vi "AMZ_S3_APIHLP_Parse NotificationConfiguration.vi"(8 "error in (no error)":errorcluster, 10 "Response body":string) -> (0 "error out":errorcluster, 3 "NotificationConfiguration":T1)   [LabVIEW 2015, in "LV Interface for Amazon S3.lvlib"]
uses:
  LV Interface for Amazon S3.lvlib
  Typedefs/AMZ_S3_NotificationConfiguration.ctl
  Typedefs/AMZ_S3_CompleteTopicConfiguration.ctl
  Typedefs/AMZ_S3_Event.ctl
  Typedefs/AMZ_S3_FilterRule.ctl
  Typedefs/AMZ_S3_CloudFunctionConfiguration.ctl
  Typedefs/AMZ_S3_QueueConfiguration.ctl
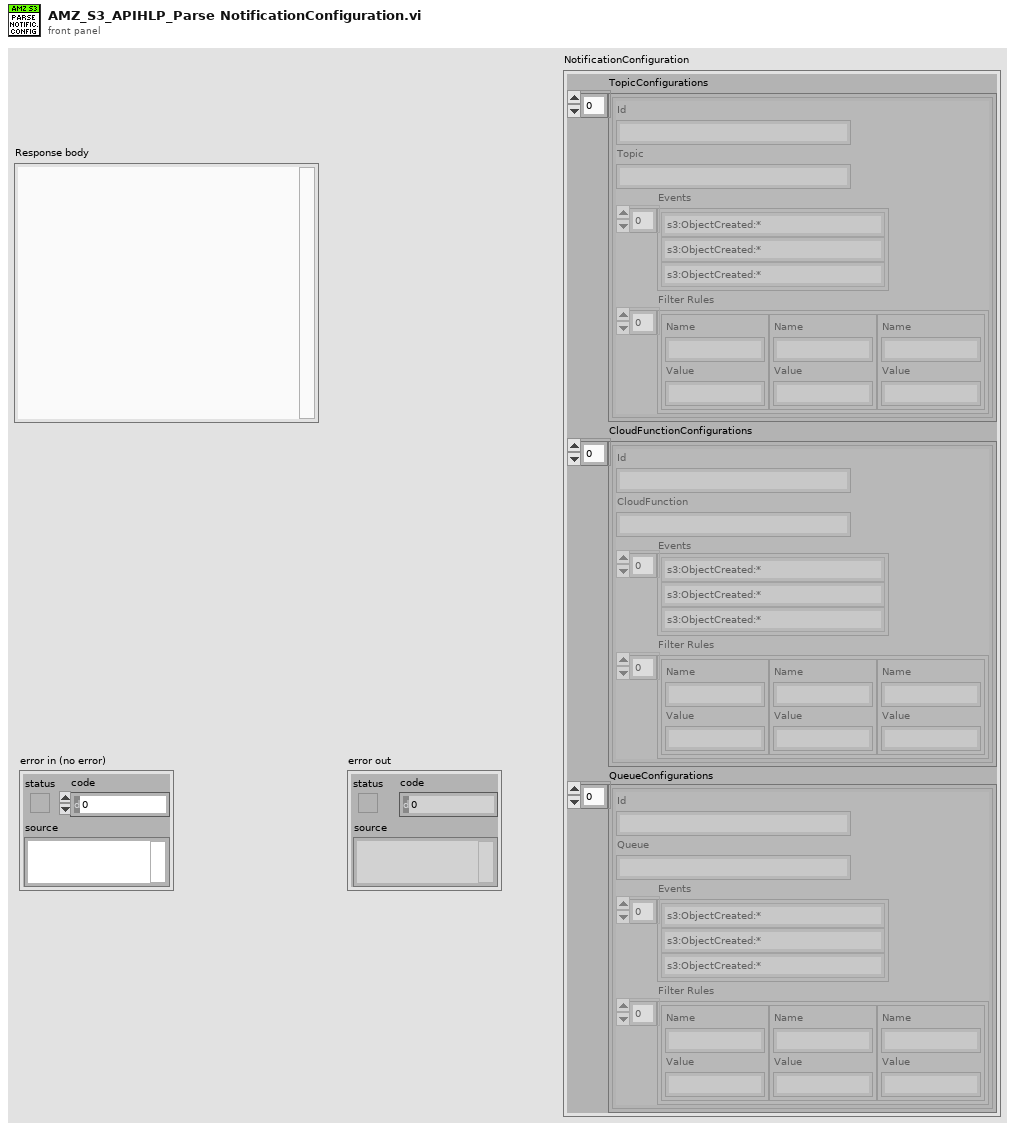
[diagram p1: front panel]
types:
  T1 = typedef "LV Interface for Amazon S3.lvlib/AMZ_S3_NotificationConfiguration.ctl" = cluster{"TopicConfigurations":T2[], "CloudFunctionConfigurations":T5[], "QueueConfigurations":T6[]}
  T2 = typedef "LV Interface for Amazon S3.lvlib/AMZ_S3_CompleteTopicConfiguration.ctl" = cluster{"Id":string, "Topic":string, "Events":T3[], "Filter Rules":T4[]}
  T3 = typedef "LV Interface for Amazon S3.lvlib/AMZ_S3_Event.ctl" = enum16{"s3:ObjectCreated:*", "s3:ObjectCreated:Put", "s3:ObjectCreated:Post", "s3:ObjectCreated:Copy", "s3:ObjectCreated:CompleteMultipartUpload", "s3:ObjectRemoved:*", "s3:ObjectRemoved:Delete", "s3:ObjectRemoved:DeleteMarkerCreated", "s3:ReducedRedundancyLostObject"}
  T4 = typedef "LV Interface for Amazon S3.lvlib/AMZ_S3_FilterRule.ctl" = cluster{"Name":string, "Value":string}
  T5 = typedef "LV Interface for Amazon S3.lvlib/AMZ_S3_CloudFunctionConfiguration.ctl" = cluster{"Id":string, "CloudFunction":string, "Events":T3[], "Filter Rules":T4[]}
  T6 = typedef "LV Interface for Amazon S3.lvlib/AMZ_S3_QueueConfiguration.ctl" = cluster{"Id":string, "Queue":string, "Events":T3[], "Filter Rules":T4[]}
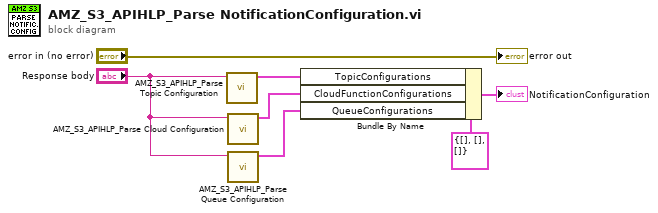
[diagram p0: block diagram]
diagram:
  n1 = call "AMZ_S3_APIHLP_Parse Topic Configuration.vi"("Response body"="Response body") -> ("Topic Configurations"=w3:T2[])  [unwired: 10 in]
  n2 = call "AMZ_S3_APIHLP_Parse Cloud Configuration.vi"("Response body"="Response body") -> ("Cloud Function Configurations"=w5:T5[])  [unwired: 10 in]
  n3 = call "AMZ_S3_APIHLP_Parse Queue Configuration.vi"("Response body"="Response body") -> ("Queue Configurations"=w1:T6[])  [unwired: 10 in]
  n4 = Bundle By Name(cluster=T1 {"TopicConfigurations"=[], "CloudFunctionConfigurations"=[], "QueueConfigurations"=[]} ("NotificationConfiguration"), "TopicConfigurations"=w3, "CloudFunctionConfigurations"=w5, "QueueConfigurations"=w1) -> (→"NotificationConfiguration":T1)
  "error out" <- "error in (no error)"
